vi "MDOSettings Dialog.vi"(8 "error in (no error)":errorcluster, 11 "Configuration in":T2 {"Hardware Configuration"."SyncMode" items=["INTERNAL"=0, "EXTERNAL_MASTER"=1, "DI_SYN1_RISE"=2, "DI_SYN1_FALL"=3, "DI_SYN2_RISE"=6, "DI_SYN2_FALL"=7]}) -> (0 "error out":errorcluster, 2 "UI Refresh Needed?":bool, 3 "Configuration out":T2 {"Hardware Configuration"."SyncMode" items=["INTERNAL"=0, "EXTERNAL_MASTER"=1, "DI_SYN1_RISE"=2, "DI_SYN1_FALL"=3, "DI_SYN2_RISE"=6, "DI_SYN2_FALL"=7]})   [LabVIEW 2020]
doc: "Dialog for selecting user specified settings."
uses:
  controls/MDOUser Specified Data.ctl
  controls/MDOHW Configuration.ctl
  controls/MDONew Data Behavior.ctl
  controls/Acquire_Type.ctl
panel:
  in  "Current_FIR_filter":bool=TRUE
  in  "Trigger Type":enum16{"No trigger", "Rise", "Fall"}(ring)=enum."Rise"
  in  "Data_save_directory":path=path "C:/Users/User/Desktop/test"
  in  "Acquire Type":T1
  in  "Cancel Button":bool
  in  "OK Button":bool
  # "Настройки"
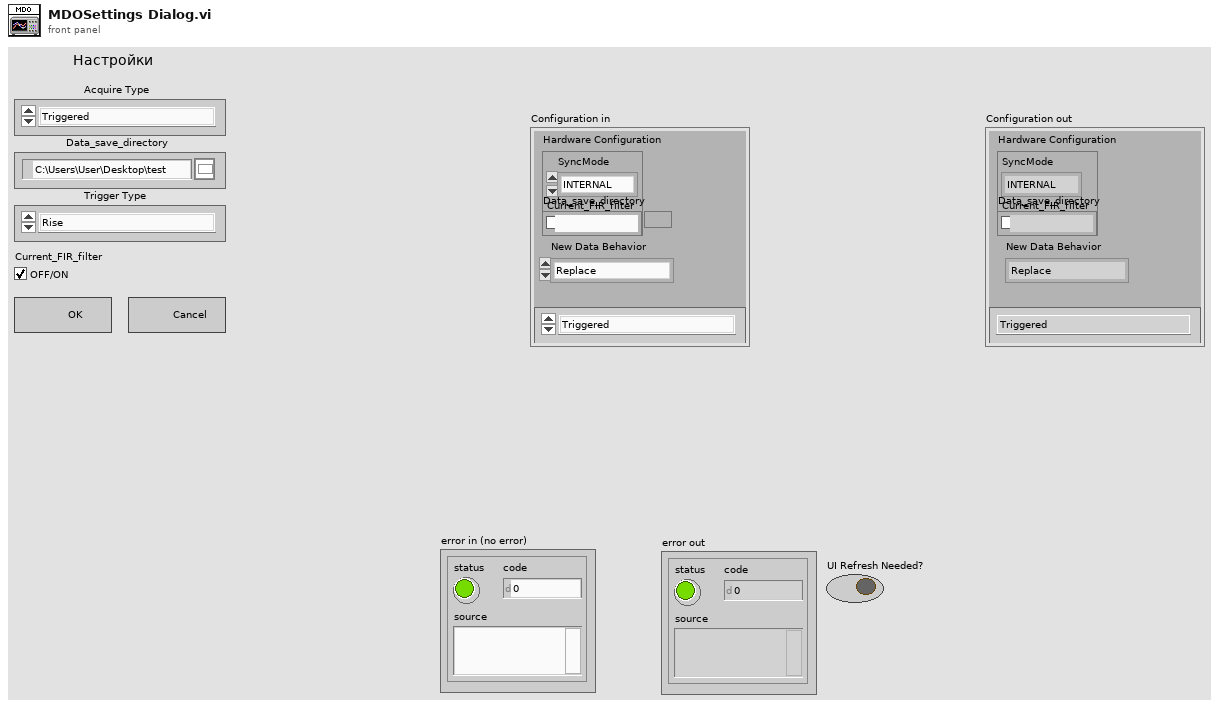
[diagram p1: front panel]
types:
  T1 = typedef "Acquire_Type.ctl" = enum16{"Triggered", "Continues"}
  T2 = typedef "MDOUser Specified Data.ctl" = cluster{"Hardware Configuration":T3, "New Data Behavior":T4, "Acquire Type":T1, "Data_save_directory":path}
  T3 = typedef "MDOHW Configuration.ctl" = cluster{"SyncMode":u32, "Current_FIR_filter":bool}
  T4 = typedef "MDONew Data Behavior.ctl" = enum16{"Replace", "Overlay", "Append"}
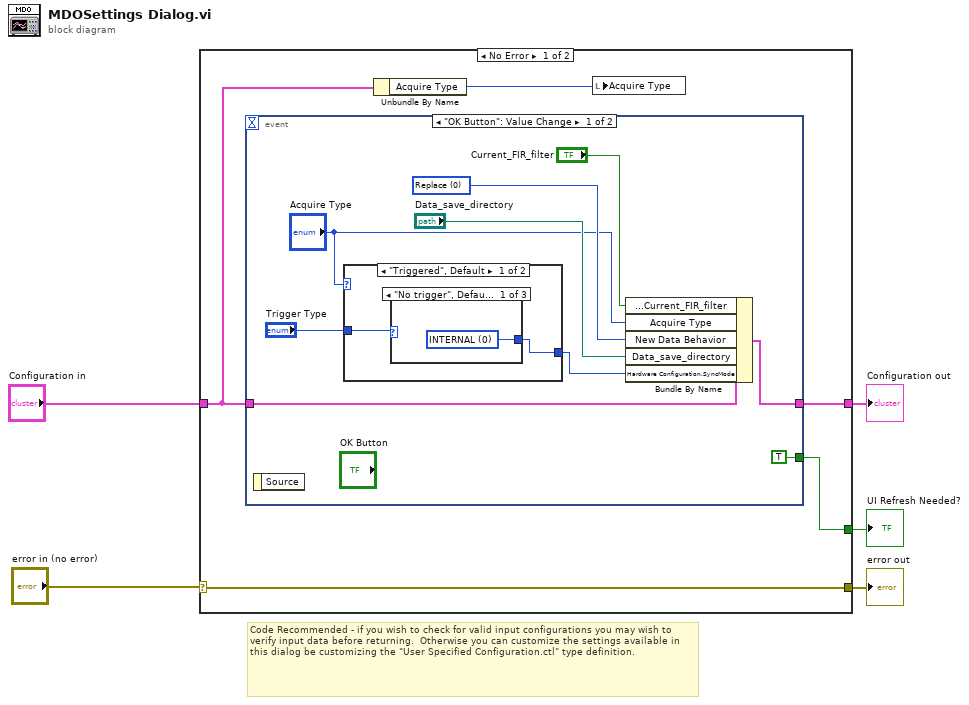
[diagram p0: block diagram]
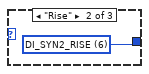
[diagram p2: hidden frame]
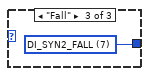
[diagram p3: hidden frame]
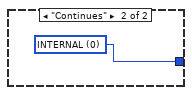
[diagram p4: hidden frame]
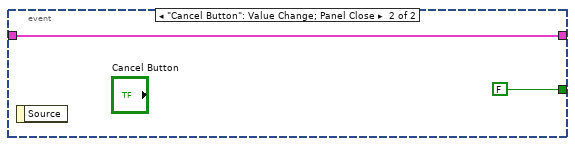
[diagram p5: hidden frame]
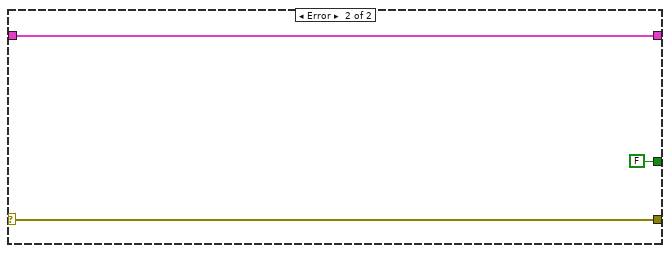
[diagram p6: hidden frame]
diagram:
  # "Code Recommended - if you wish to check for valid input configurations you may wish to verify input data before returning.  Otherwise you can customize the settings available in this dialog be customizing the \"User Specified Configuration.ctl\" type definition."
  n1 = case shown="No Error" "error in (no error)" {
    selector: "error in (no error)" -> [w10 w30]
    tunnel: [w10 w30] -> w4
    tunnel: "Configuration in" -> [w8 w29]
    tunnel: [w9 w29] -> w2
    tunnel: [w7 FALSE ("UI Refresh Needed?")] -> w1
    frame No Error {
      n2 = event shown="[0] \"OK Button\": Value Change" {
        selector: _ -> [_ _]
        dyn-events: _ -> [_ _]
        timeout: _ -> [_ _]
        tunnel: [w16 w27] -> w9
        tunnel: w8 -> [w19 w27]
        tunnel: [TRUE ("UI Refresh Needed?") FALSE ("UI Refresh Needed?")] -> w7
        event "OK Button": Value Change {
          w18 = u16 0 items=["Replace", "Overlay", "Append"] ("New Data Behavior")
          n3 = event-data() -> ()  [unwired: 1 in, 1 out]
          n4 = case shown="\"Triggered\", Default" "Acquire Type" {
            tunnel: "Trigger Type" -> [w21 _]
            tunnel: [w20 w25] -> w12
            frame "Triggered", Default {
              n5 = case shown="\"No trigger\", Default" w21 {
                tunnel: [w22 w23 w24] -> w20
                frame "No trigger", Default {
                  w22 = u32 0 items=["INTERNAL"=0, "EXTERNAL_MASTER"=1, "DI_SYN1_RISE"=2, "DI_SYN1_FALL"=3, "DI_SYN2_RISE"=6, "DI_SYN2_FALL"=7] ("SyncMode")
                }
                frame "Rise" {
                  w23 = u32 6 items=["INTERNAL"=0, "EXTERNAL_MASTER"=1, "DI_SYN1_RISE"=2, "DI_SYN1_FALL"=3, "DI_SYN2_RISE"=6, "DI_SYN2_FALL"=7] ("SyncMode")
                }
                frame "Fall" {
                  w24 = u32 7 items=["INTERNAL"=0, "EXTERNAL_MASTER"=1, "DI_SYN1_RISE"=2, "DI_SYN1_FALL"=3, "DI_SYN2_RISE"=6, "DI_SYN2_FALL"=7] ("SyncMode")
                }
              }
            }
            frame "Continues" {
              w25 = u32 0 items=["INTERNAL"=0, "EXTERNAL_MASTER"=1, "DI_SYN1_RISE"=2, "DI_SYN1_FALL"=3, "DI_SYN2_RISE"=6, "DI_SYN2_FALL"=7] ("SyncMode")
            }
          }
          n6 = Bundle By Name(cluster=w19, "Hardware Configuration.Current_FIR_filter"="Current_FIR_filter", "Acquire Type"="Acquire Type", "New Data Behavior"=w18, "Data_save_directory"="Data_save_directory", "Hardware Configuration.SyncMode"=w12) -> (w16:T2)
        }
        event "Cancel Button": Value Change; Panel Close {
          n7 = event-data() -> ()  [unwired: 1 in, 1 out]
        }
      }
      n8 = Unbundle By Name(w8) -> ("Acquire Type"=w6:T1)
      n9 = local write "Acquire Type"(w6) -> ()
    }
    frame Error {
    }
  }
  "UI Refresh Needed?" <- w1
  "error out" <- w4
  "Configuration out" <- w2
